vi "Remove Icon Template.vi"(8 "error in (no error)":errorcluster, 11 "VI Ref":refnum<vi>) -> (0 "error out":errorcluster, 2 "Save?":bool, 3 "VI Ref out":refnum<vi>)   [LabVIEW 2020, in "Code Cleanup.lvlib"]
uses:
  Code Cleanup.lvlib
  <vilib>/LabVIEW Icon API/lv_icon/Classes/Icon Framework/Icon Framework.lvclass
  <vilib>/LabVIEW Icon API/lv_icon/Classes/Icon/Icon.lvclass
  <vilib>/LabVIEW Icon API/LabVIEW Icon API.lvlib
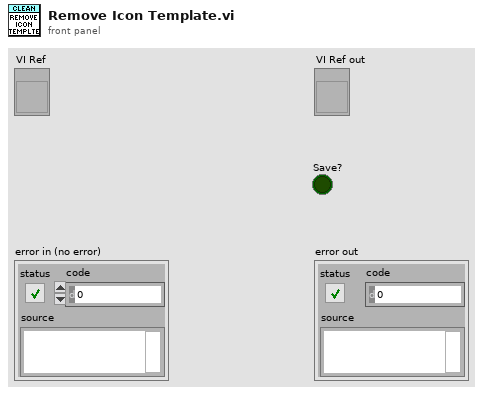
[diagram p1: front panel]
types:
  T1 = typedef "Layer.ctl" = cluster{"LayerIcon":picture, "LayerName":string, "Opacity":u8, "Visibility?":bool}
  T2 = typedef "imagedata.ctl" = cluster{"image type":i32, "image depth":i32, "image":u8[], "mask":u8[], "colors":u32[], "Rectangle":cluster{"left":i16, "top":i16, "right":i16, "bottom":i16}}
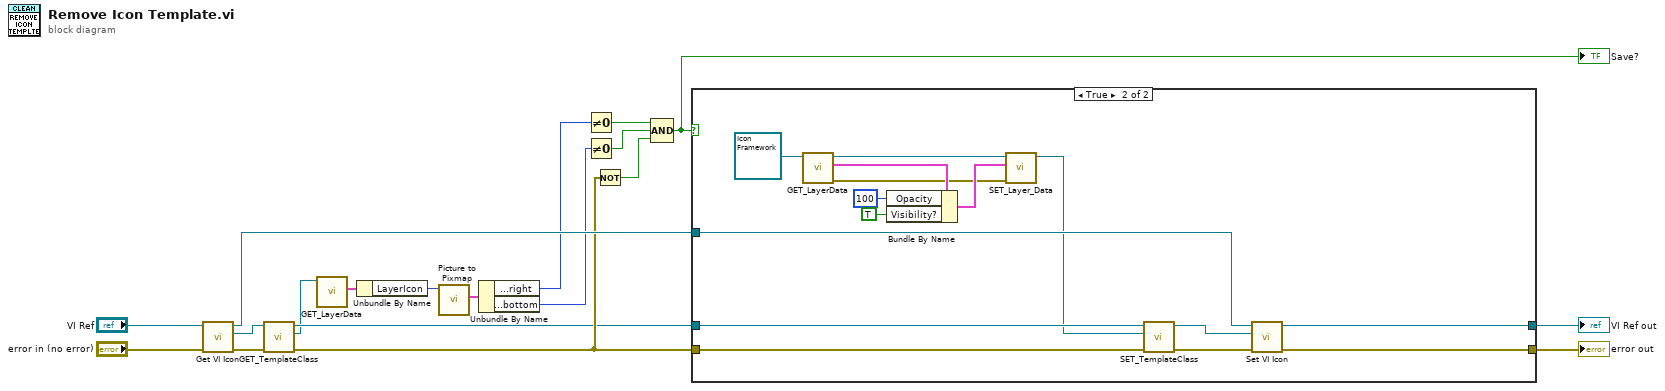
[diagram p0: block diagram]
diagram:
  n1 = call <vilib>:"Get VI Icon.vi"("error in (no error)"="error in (no error)", "VI Refnum in"="VI Ref") -> ("error out"=w14:errorcluster, "Icon"=w12:refnum<class "Icon.lvclass">, "VI Refnum out"=w17:refnum<vi>)  [unwired: 7 in]
  n2 = call-dynamic "GET_TemplateClass.vi"("error in (no error)"=w14, "Icon.lvclass in"=w12) -> ("error out"=w13:errorcluster, "Icon Framework.lvclass"=w10:refnum<class "Icon Framework.lvclass">, "Icon.lvclass out"=w11:refnum<class "Icon.lvclass">)  [unwired: 7 in]
  n3 = call-dynamic "GET_LayerData.vi"("Layer.lvclass in"=w10) -> ("Data"=w9:T1)  [unwired: 6 in, 4 out]
  n4 = Unbundle By Name(w9) -> ("LayerIcon"=w7:picture)
  n5 = call <vilib>:"Picture to Pixmap.vi"("picture"=w7) -> ("image data"=w8:T2)  [unwired: 9 in, 1 out]
  n6 = Unbundle By Name(w8) -> ("Rectangle.right"=w6:i16, "Rectangle.bottom"=w5:i16)
  n7 = Not Equal To 0?(x=w6) -> (x != 0?=w16:bool)
  n8 = Not Equal To 0?(x=w5) -> (x != 0?=w15:bool)
  n9 = Not(x=w13) -> (.not. x?=w18:bool)
  n10 = Compound Arithmetic op=AND(w16, w15, w18) -> (w19:bool)
  "Save?" <- w19
  n11 = case shown="True" w19 {
    tunnel: w13 -> [w21 w35]
    tunnel: [w21 w23] -> w3
    tunnel: [w20 w22] -> w2
    tunnel: w17 -> [w20 w36]
    tunnel: w11 -> [_ w34]
    frame False {
    }
    frame True {
      n12 = call-dynamic "GET_LayerData.vi"("Layer.lvclass in"=refnum<class "Icon Framework.lvclass"> refnum ("Icon Framework.lvclass")) -> ("error out"=w28:errorcluster, "Data"=w29:T1, "Layer.lvclass out"=w30:refnum<class "Icon Framework.lvclass">)  [unwired: 6 in, 2 out]
      n13 = Bundle By Name(cluster=w29, "Opacity"=u8 100, "Visibility?"=TRUE) -> (w31:T1)
      n14 = call-dynamic "SET_Layer_Data.vi"("error in (no error)"=w28, "Data"=w31, "Layer.lvclass in"=w30) -> ("Layer.lvclass out"=w24:refnum<class "Icon Framework.lvclass">)  [unwired: 7 in, 1 out]
      n15 = call-dynamic "SET_TemplateClass.vi"("error in (no error)"=w35, "Icon Framework.lvclass"=w24, "Icon.lvclass in"=w34) -> ("error out"=w33:errorcluster, "Icon.lvclass out"=w32:refnum<class "Icon.lvclass">)  [unwired: 7 in]
      n16 = call <vilib>:"Set VI Icon.vi"("error in (no error)"=w33, "Icon"=w32, "VI Refnum in"=w36) -> ("error out"=w23:errorcluster, "VI Refnum out"=w22:refnum<vi>)  [unwired: 7 in]
    }
  }
  "error out" <- w3
  "VI Ref out" <- w2
